vi "shooterPID.vi"(1 "rpmTarget":dbl, 2 "CounterDevRef":T1) -> (7 "output":dbl format="%.2f")   [LabVIEW 2012]
uses:
  <vilib>/Rock Robotics/WPI/Counter/WPI_CounterDevRef.ctl
  <vilib>/Rock Robotics/SystemInterfaces/Counter/FPGA_CounterCtrSystemIndex.ctl
  <vilib>/addons/control/pid/pid.llb/PID (DBL).vi
  <vilib>/addons/control/pid/NI_PID_pid.lvlib
panel:
  out "pidGains":T3={"proportional gain (Kc)"=1.0, "integral time (Ti, min)"=0.01, "derivative time (Td, min)"=0.0} {"derivative time (Td, min)" format="%.3f"; "integral time (Ti, min)" format="%.3f"; "proportional gain (Kc)" format="%.3f"}
  out "withinRangeMotor1":bool
  in  "rpmRangeMotor1":dbl
  out "rpmCurrentMotor1":dbl
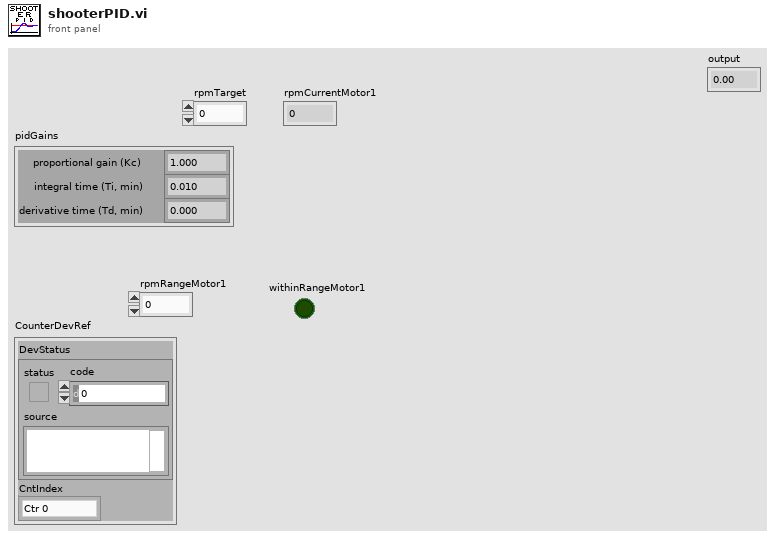
[diagram p1: front panel]
types:
  T1 = typedef "WPI_CounterDevRef.ctl" = cluster{"DevStatus":errorcluster, "CntIndex":T2}
  T2 = typedef "FPGA_CounterCtrSystemIndex.ctl" = enum8{"Ctr 0", "Ctr 1", "Ctr 2", "Ctr 3", "Ctr 4", "Ctr 5", "Ctr 6", "Ctr 7", "Invalid"}
  T3 = cluster{"proportional gain (Kc)":dbl, "integral time (Ti, min)":dbl, "derivative time (Td, min)":dbl}
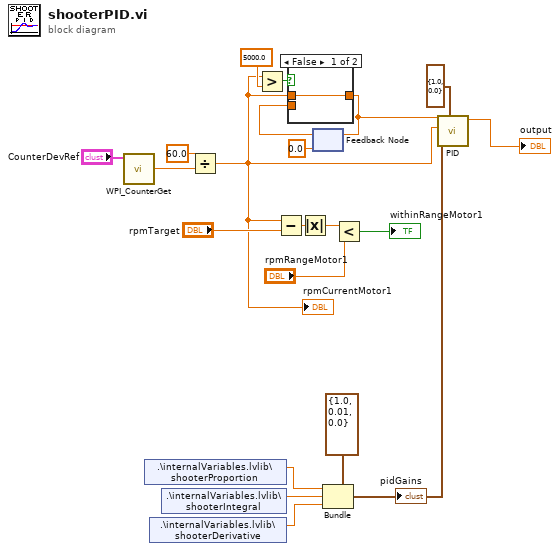
[diagram p0: block diagram]
diagram:
  n1 = call <vilib>:"WPI_CounterGet.vi"("CounterDevRef in"="CounterDevRef") -> ("Period (sec)"=w20:dbl)  [unwired: 5 in, 5 out]
  n2 = shared-variable ".\\internalVariables.lvlib\\shooterProportion"() -> (w5:dbl)  [unwired: 1 in, 1 out]
  n3 = shared-variable ".\\internalVariables.lvlib\\shooterDerivative"() -> (w3:dbl)  [unwired: 1 in, 1 out]
  n4 = shared-variable ".\\internalVariables.lvlib\\shooterIntegral"() -> (w4:dbl)  [unwired: 1 in, 1 out]
  n5 = Divide(x=60.0, y=w20) -> (x/y=w1:dbl)
  "rpmCurrentMotor1" <- w1
  n6 = Greater?(x=w1, y=5000.0) -> (0:w11:bool)
  n7 = Subtract(x=w1, y="rpmTarget") -> (x-y=w17:dbl)
  n8 = Absolute Value(x=w17) -> (abs(x)=w16:dbl)
  n9 = feedback #1(0.0 ("rpmTarget")) -> (w9:dbl)
  n10 = case shown="False" w11 {
    tunnel: w1 -> [w22 _]
    tunnel: [w22 w23] -> w8
    tunnel: w9 -> [_ w23]
    frame False {
    }
    frame True {
    }
  }
  n11 = feedback-in #1(w8) -> ()
  n12 = Bundle(cluster=T3 {"proportional gain (Kc)"=1.0, "integral time (Ti, min)"=0.01, "derivative time (Td, min)"=0.0} ("pidGains"), "proportional gain (Kc)"=w5, "integral time (Ti, min)"=w4, "derivative time (Td, min)"=w3) -> (w2:T3)
  "pidGains" <- w2
  n13 = Less?(x=w16, y="rpmRangeMotor1") -> (x < y?=→"withinRangeMotor1":bool)
  n14 = call-poly <vilib>:"PID.vi"("output range"=cluster{"output high":dbl, "output low":dbl} {"output high"=1.0, "output low"=0.0}, "PID gains"=w2, "process variable"=w1, "setpoint"=w8) -> ("output"=→"output":dbl)  [unwired: 6 in, 1 out]
